vi "Extract.vi"(8 "error in (no error)":errorcluster, 10 "AbstractData in":refnum<class "AbstractData.lvclass">, 11 "AbstractExtractor2D in":refnum<class "AbstractExtractor2D.lvclass">) -> (0 "error out":errorcluster, 3 "AbstractExtractor2D out":refnum<class "AbstractExtractor2D.lvclass">)   [LabVIEW 2014, in "AbstractExtractor2D.lvclass"]
uses:
  AbstractExtractor2D.lvclass
  Model/Data/AbstractData/AbstractData.lvclass
  Model/Data/Data2D/Data2D.lvclass
  AbstractExtractor/AbstractExtractor.lvclass
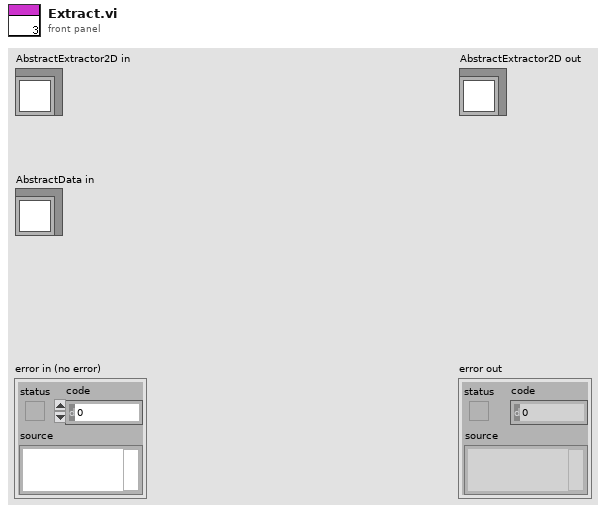
[diagram p1: front panel]
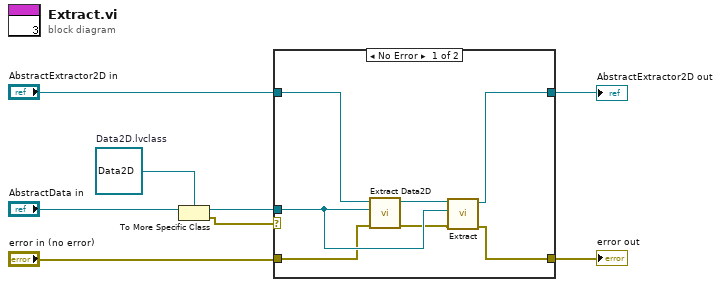
[diagram p0: block diagram]
diagram:
  w6 = refnum<class "Data2D.lvclass"> refnum  # Data2D.lvclass
  n1 = To More Specific Class(target class=w6, reference="AbstractData in") -> (specific class reference=w7:refnum<class "Data2D.lvclass">, error out=w8:errorcluster)  [unwired: 1 in]
  n2 = case shown="No Error" w8 {
    tunnel: w7 -> [w11 _]
    tunnel: "error in (no error)" -> [w10 w17]
    tunnel: [w15 w17] -> w4
    tunnel: "AbstractExtractor2D in" -> [w12 w16]
    tunnel: [w14 w16] -> w5
    frame No Error {
      n3 = call-dynamic "Extract Data2D.vi"("error in (no error)"=w10, "Data2D in"=w11, "AbstractExtractor2D in"=w12) -> ("error out"=w9:errorcluster, "AbstractExtractor2D out"=w13:refnum<class "AbstractExtractor2D.lvclass">)  [unwired: 7 in]
      n4 = call-parent "Extract.vi"("error in (no error)"=w9, "AbstractData in"=w11, "AbstractExtractor in"=w13) -> ("error out"=w15:errorcluster, "AbstractExtractor out"=w14:refnum<class "AbstractExtractor2D.lvclass">)  [unwired: 7 in]
    }
    frame Error {
    }
  }
  "error out" <- w4
  "AbstractExtractor2D out" <- w5
